vi "rti.global.vi"() -> ()   [LabVIEW 2019]
panel:
  in  "sm-main-center-tol":u64=5580754
  in  "sm-main-center-hs-thres":u64=55807545
  in  "io.encoder-center":u64=68719476735
  in  "io.cloud-enable":bool
  in  "sm.cloud-timeout (ms)":u32=300000
  in  "sm.encoder-no-error":u16=1025 format="%x"
  in  "sm.az-timeout (ms)":u32=300000
  in  "sm.rev-dly (ms)":u32=2000
  in  "sm.main-pos-hs-thres":fxp<+/-,32,2>=0.20000000018626451
  in  "sm.main-pos-tol":fxp<+/-,32,2>=0.049999999813735485
  in  "io.encoder-negate":bool
  in  "io.home-pos":fxp<+/-,32,2>
  in  "io.encoder-step":u64=10000
  in  "io.encoder-ref":u64
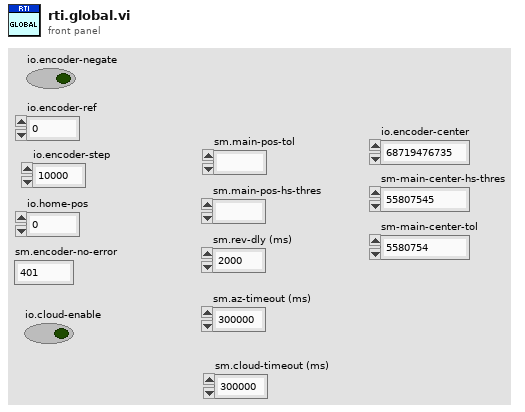
[diagram p1: front panel]
diagram:
